vi "Calculate desired heading.vi"(0 "Arbiter Array":dbl[](array[numeric])) -> (1 "Desired Heading":i32, 2 "Desired Velocity":i32)   [LabVIEW 2012]
doc: "This VI accepts a 1D arbiter array as an input. It calculate the max value of the array and its index. The desired heading is calculated by transforming the index value such that and index of 44 represents a heading of 0 degrees. The heading output is +/- 45 degrees where positive degrees are to starboard in the local corrdinate system of the tug. The velocity output is between +/- 9."
panel:
  out "Waveform Graph":dbl[](graph)
  out "max index(es)":i32
  out "max value":dbl
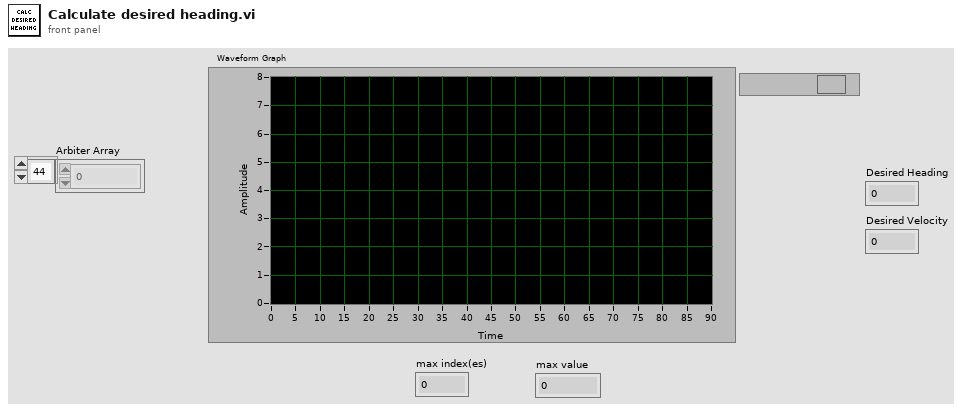
[diagram p1: front panel]
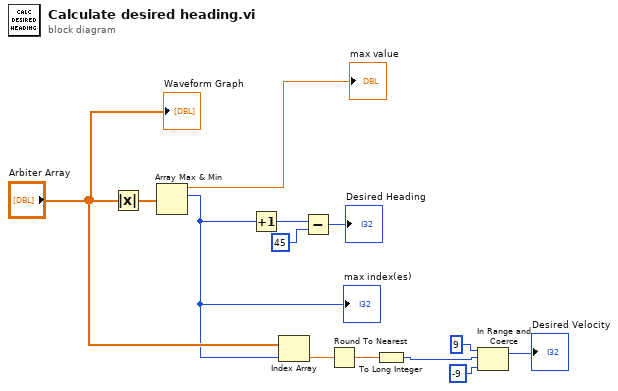
[diagram p0: block diagram]
diagram:
  n1 = Absolute Value(x="Arbiter Array") -> (abs(x)=w9:dbl[])
  n2 = Array Max & Min(array=w9) -> (max value=→"max value":dbl, max index (indices)=w7:i32)  [unwired: 2 out]
  "max index(es)" <- w7
  n3 = Increment(x=w7) -> (x+1=w12:i32)
  n4 = Index Array(array="Arbiter Array", index=w7) -> (element=w3:dbl)
  n5 = Subtract(x=w12, y=45) -> (x-y=→"Desired Heading":i32)
  n6 = Round To Nearest(number=w3) -> (nearest integer value=w2:dbl)
  n7 = To Long Integer(number=w2) -> (32bit integer=w1:i32)
  n8 = In Range and Coerce(upper limit=9, x=w1, lower limit=-9) -> (coerced(x)=→"Desired Velocity":i32)  [unwired: 1 out]
  "Waveform Graph" <- "Arbiter Array"
